vi "Test Alarm API.vi"() -> ()   [LabVIEW 2018]
uses:
  Alarm.lvclass
  Alarm.lvclass/Alarm.ctl
  Get Alarm Reason.vi
panel:
  out "error out":errorcluster
  in  "Alarm Reason":string="fire"
  in  "Alarm in":bool=TRUE
  out "Alarm Reasons":string[](array[string])
  in  "Activate Alarm":bool caption="Open Door"
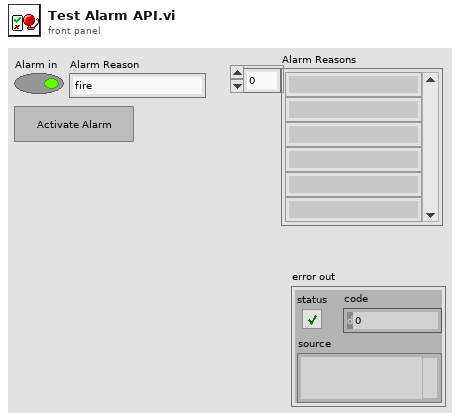
[diagram p1: front panel]
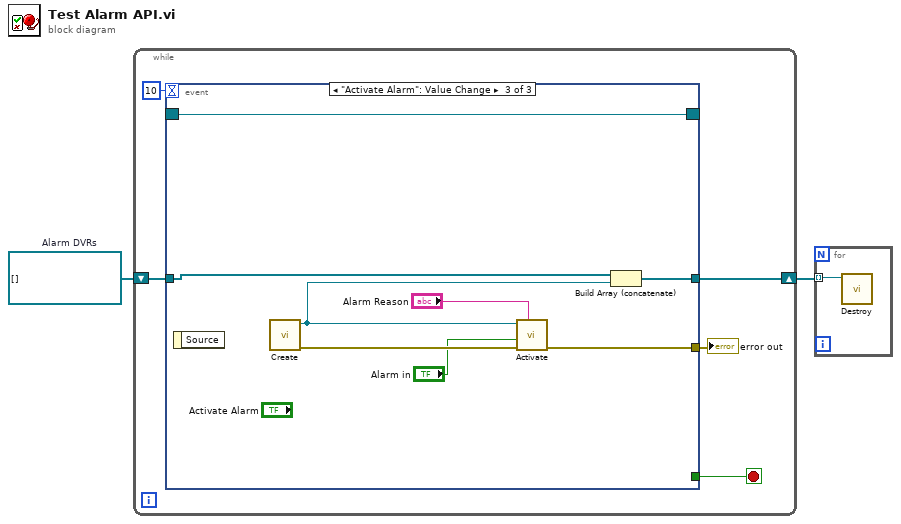
[diagram p0: block diagram]
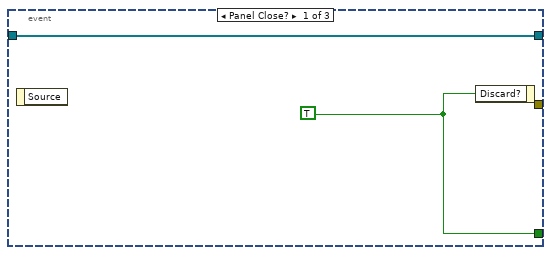
[diagram p2: hidden frame]
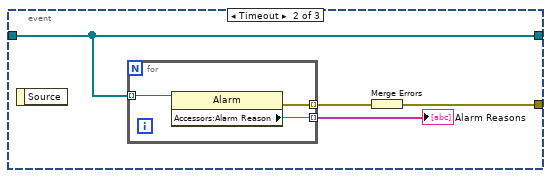
[diagram p3: hidden frame]
diagram:
  w2 = refnum<data-value>[] []  # Alarm DVRs
  n1 = while {
    shift-right: [w5] -> w1
    shift-left: w2 -> [w6]
    stop <- w7 stop-if-true
    n2 = event shown="[2] \"Activate Alarm\": Value Change" {
      selector: _ -> [_ _ w22]
      dyn-events: [_ _ w22] -> _
      timeout: 10 -> [_ _ _]
      tunnel: [w9 _ _] -> w7
      tunnel: w6 -> [w8 w13 w24]
      tunnel: [w8 w13 w23] -> w5
      tunnel: [_ w10 w17] -> w3
      event Panel Close? {
        w9 = TRUE ("Discard?")
        n3 = event-data() -> ()  [unwired: 1 in, 1 out]
        n4 = event-data("Discard?"=w9) -> ()  [unwired: 1 in, 1 out]
      }
      event Timeout {
        n5 = event-data() -> ()  [unwired: 1 in, 1 out]
        n6 = for {
          tunnel: w13 -> [w16] mode=indexing
          tunnel: [w15] -> w12 mode=indexing
          tunnel: [w14] -> w11 mode=indexing
          n7 = property class="Alarm"(reference=w16) -> (error out=w14:errorcluster, "Accessors:Alarm Reason"=w15:string)  [unwired: 1 in, 1 out]
        }
        "Alarm Reasons" <- w12
        n8 = Merge Errors(w11) -> (w10:errorcluster)
      }
      event "Activate Alarm": Value Change {
        n9 = event-data() -> ()  [unwired: 1 in, 1 out]
        n10 = call "Create.vi"() -> ("error out"=w21:errorcluster, "Alarm DVR"=w18:refnum<data-value>)  [unwired: 10 in]
        n11 = call "Activate.vi"("Alarm Reason"="Alarm Reason", "error in (no error)"=w21, "Alarm in"="Alarm in", "Data Value Reference in"=w18) -> ("error out"=w17:errorcluster)  [unwired: 7 in]
        n12 = Build Array (concatenate)(w24, w18) -> (w23:refnum<data-value>[])
      }
    }
    "error out" <- w3
  }
  n13 = for {
    tunnel: w1 -> [w25] mode=indexing
    n14 = call "Destroy.vi"("Alarm DVR"=w25) -> ()  [unwired: 10 in, 1 out]
  }
